vi "Actor Core.vi"(8 "error in":errorcluster, 11 "Nested in":refnum<class "UI Actor.lvclass">) -> (0 "error out":errorcluster, 3 "Actor out":refnum<class "Actor.lvclass">)   [LabVIEW 2020, in "UI Actor.lvlib" / "UI Actor.lvclass"]
doc: "(<B>Filename</B>: Actor Framework.lvlib:Actor.lvclass:Actor Core.vi)\n\nReceives messages to the actor, reacts to them, and initiates any error handling that may shut the actor down.\n\nDescendant classes may override this VI to append parallel tasks for the actor to complete while it handles messages. Overrides use the Call Parent Method node."
uses:
  UI Actor.lvclass
  C:/Program Files (x86)/National Instruments/LabVIEW 2020/vi.lib/ActorFramework/Actor/Actor.lvclass
  <vilib>/ActorFramework/Actor/Actor.lvclass
  <vilib>/ActorFramework/Actor/Actor.lvclass/Actor.ctl
  <vilib>/ActorFramework/Message Enqueuer/Message Enqueuer.lvclass/Message Enqueuer.ctl
  UI Actor.lvclass/UI Actor.ctl
  UI Actor Messages/Set Com Port Msg/Set Com Port Msg.lvclass/Set Com Port Msg.ctl
  UI Actor Messages/Read ADC_UI Actor Msg/Read ADC_UI Actor Msg.lvclass/Read ADC_UI Actor Msg.ctl
  UI Actor Messages/Get Port Status_UI Actor Msg/Get Port Status_UI Actor Msg.lvclass/Get Port Status_UI Actor Msg.ctl
  UI Actor Messages/Set Port Status_UI Actor Msg/Set Port Status_UI Actor Msg.lvclass/Set Port Status_UI Actor Msg.ctl
  UI Actor Messages/Get Pin Status_UI Actor Msg/Get Pin Status_UI Actor Msg.lvclass/Get Pin Status_UI Actor Msg.ctl
  UI Actor Messages/Set Pin Status_UI Actor Msg/Set Pin Status_UI Actor Msg.lvclass/Set Pin Status_UI Actor Msg.ctl
  UI Actor Messages/Set CH Msg/Set CH Msg.lvclass/Set CH Msg.ctl
  UI Actor Messages/Set Pin Msg/Set Pin Msg.lvclass/Set Pin Msg.ctl
  UI Actor Messages/Set valor PIN Msg/Set valor PIN Msg.lvclass/Set valor PIN Msg.ctl
  <vilib>/ActorFramework/Message Enqueuer/Init from Existing Queue.vi
  <vilib>/ActorFramework/Message Enqueuer/Enqueue.vi
  <vilib>/ActorFramework/Stop Msg/Stop Msg.lvclass
  C:/Program Files (x86)/National Instruments/LabVIEW 2020/vi.lib/ActorFramework/Message/Message.lvclass
  UI Actor Messages/Set Com Port Msg/Set Com Port Msg.lvclass
  UI Actor Messages/Read ADC_UI Actor Msg/Read ADC_UI Actor Msg.lvclass
  UI Actor Messages/Get Port Status_UI Actor Msg/Get Port Status_UI Actor Msg.lvclass
  UI Actor Messages/Set Port Status_UI Actor Msg/Set Port Status_UI Actor Msg.lvclass
  UI Actor Messages/Get Pin Status_UI Actor Msg/Get Pin Status_UI Actor Msg.lvclass
  UI Actor Messages/Set Pin Status_UI Actor Msg/Set Pin Status_UI Actor Msg.lvclass
  UI Actor Messages/Set CH Msg/Set CH Msg.lvclass
  UI Actor Messages/Set Pin Msg/Set Pin Msg.lvclass
  UI Actor Messages/Set valor PIN Msg/Set valor PIN Msg.lvclass
  <vilib>/ActorFramework/Message Priority Queue/Priority Enqueue.vi
  <vilib>/Instr/_visa.llb/VISA Configure Serial Port (Instr).vi
  <vilib>/ActorFramework/Message Enqueuer/Message Enqueuer.lvclass
panel:
  in  "Byte 0":string(combo)
  in  "Byte 1":string(combo)
  in  "Valor pin":string(combo)
  in  "PIN":i32
  in  "CH":i32
  out "Display":string
  in  "Set Pin Status":bool
  in  "Get Pin Status":bool
  in  "Set Port Status":bool
  in  "Get Port Status":bool
  in  "Read ADC":bool
  in  "VISA":refnum<visa-resource-name>
  in  "OK Button":bool
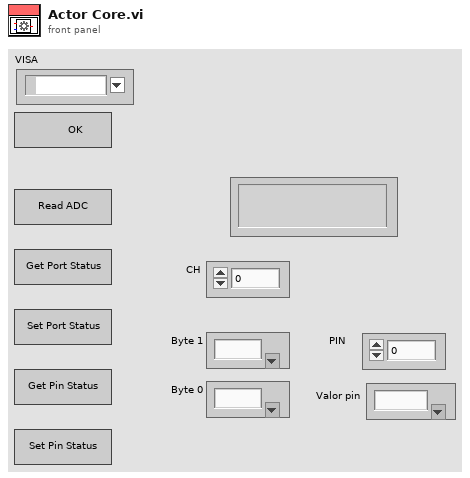
[diagram p1: front panel]
types:
  T1 = cluster{"Stop":refnum<user-event>, "Display":refnum<user-event>}
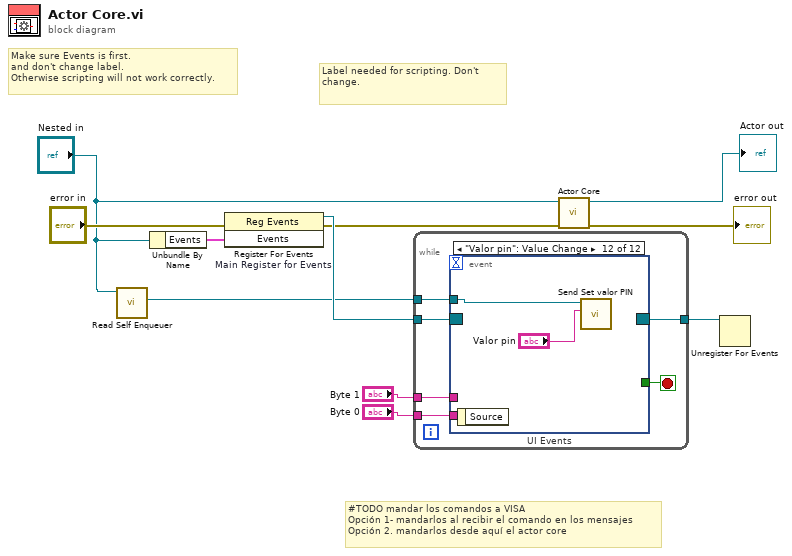
[diagram p0: block diagram]
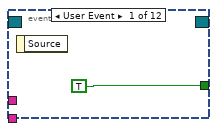
[diagram p2: hidden frame]
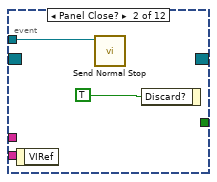
[diagram p3: hidden frame]
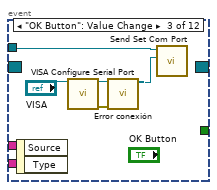
[diagram p4: hidden frame]
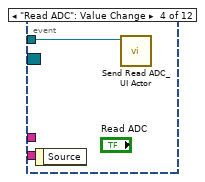
[diagram p5: hidden frame]
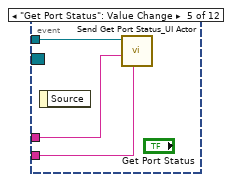
[diagram p6: hidden frame]
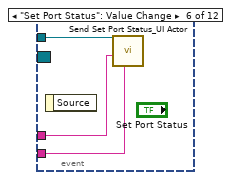
[diagram p7: hidden frame]
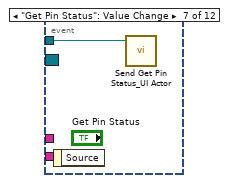
[diagram p8: hidden frame]
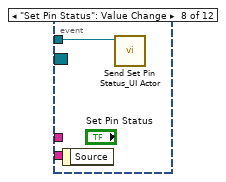
[diagram p9: hidden frame]
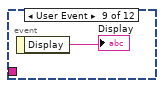
[diagram p10: hidden frame]
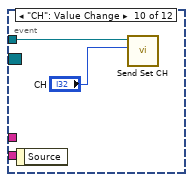
[diagram p11: hidden frame]
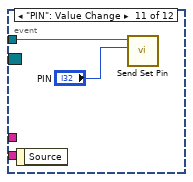
[diagram p12: hidden frame]
diagram:
  # "#TODO mandar los comandos a VISA\nOpción 1- mandarlos al recibir el comando en los mensajes\nOpción 2. mandarlos desde aquí el actor core"
  # "Label needed for scripting. Don't change."
  # "Make sure Events is first.\nand don't change label.\nOtherwise scripting will not work correctly."
  n1 = call <vilib>:"Read Self Enqueuer.vi"("Actor"="Nested in") -> ("Self Enqueuer"=w6:refnum<class "Message Enqueuer.lvclass">)  [unwired: 10 in]
  n2 = Unbundle By Name("Nested in") -> ("Events"=w8:T1)
  n3 = register-events "Main Register for Events"(error in="error in", w8) -> (reference out=w9:refnum<event-registration>, error out=w4:errorcluster)  [unwired: 1 in]
  n4 = while {
    tunnel: w9 -> [w17]
    tunnel: [w15] -> w7
    tunnel: w6 -> [w14]
    tunnel: "Byte 1" -> [w13]
    tunnel: "Byte 0" -> [w12]
    stop <- w16 stop-if-true
    n5 = event "UI Events" shown="[11] \"Valor pin\": Value Change" {
      selector: w17 -> [_ _ _ _ _ _ _ _ _ _ _ _]
      dyn-events: [_ _ _ _ _ _ _ _ _ _ _ _] -> w15
      timeout: _ -> [_ _ _ _ _ _ _ _ _ _ _ _]
      tunnel: [TRUE _ _ _ _ _ _ _ _ _ _ _] -> w16
      tunnel: w14 -> [_ w19 w25 w26 w29 w32 w33 w34 _ w37 w39 w41]
      tunnel: w13 -> [_ _ _ _ w28 w31 _ _ _ _ _ _]
      tunnel: w12 -> [_ _ _ _ w27 w30 _ _ _ _ _ _]
      event User Event {
        n6 = event-data() -> ()  [unwired: 1 in, 1 out]
      }
      event Panel Close? {
        n7 = event-data() -> ()  [unwired: 1 in, 1 out]
        n8 = call <vilib>:"Send Normal Stop.vi"("Message Enqueuer"=w19) -> ()  [unwired: 10 in, 1 out]
        n9 = event-data("Discard?"=TRUE) -> ()  [unwired: 1 in, 1 out]
      }
      event "OK Button": Value Change {
        n10 = event-data() -> ()  [unwired: 1 in, 2 out]
        n11 = call-poly "VISA Configure Serial Port"("VISA resource name"="VISA") -> ("VISA resource name out"=w22:refnum<visa-resource-name>, "error out"=w23:errorcluster)  [unwired: 13 in]
        n12 = call "Error conexión.vi"("error in (no error)"=w23, "VISA Refnum in"=w22) -> ("VISA Refnum out"=w21:refnum<visa-resource-name>)  [unwired: 9 in]
        n13 = call "Send Set Com Port.vi"("VISA resource name"=w21, "Message Enqueuer"=w25) -> ()  [unwired: 8 in, 2 out]
      }
      event "Read ADC": Value Change {
        n14 = event-data() -> ()  [unwired: 1 in, 1 out]
        n15 = call "Send Read ADC_UI Actor.vi"("Message Enqueuer"=w26) -> ()  [unwired: 9 in, 2 out]
      }
      event "Get Port Status": Value Change {
        n16 = event-data() -> ()  [unwired: 1 in, 1 out]
        n17 = call "Send Get Port Status_UI Actor.vi"("Byte 0"=w27, "Byte 1"=w28, "Message Enqueuer"=w29) -> ()  [unwired: 7 in, 2 out]
      }
      event "Set Port Status": Value Change {
        n18 = event-data() -> ()  [unwired: 1 in, 1 out]
        n19 = call "Send Set Port Status_UI Actor.vi"("Byte 0"=w30, "Byte 1"=w31, "Message Enqueuer"=w32) -> ()  [unwired: 7 in, 2 out]
      }
      event "Get Pin Status": Value Change {
        n20 = event-data() -> ()  [unwired: 1 in, 1 out]
        n21 = call "Send Get Pin Status_UI Actor.vi"("Message Enqueuer"=w33) -> ()  [unwired: 9 in, 2 out]
      }
      event "Set Pin Status": Value Change {
        n22 = event-data() -> ()  [unwired: 1 in, 1 out]
        n23 = call "Send Set Pin Status_UI Actor.vi"("Message Enqueuer"=w34) -> ()  [unwired: 9 in, 2 out]
      }
      event User Event {
        n24 = event-data() -> ("Display"=→"Display":string)  [unwired: 1 in]
      }
      event "CH": Value Change {
        n25 = event-data() -> ()  [unwired: 1 in, 1 out]
        n26 = call "Send Set CH.vi"("CH"="CH", "Message Enqueuer"=w37) -> ()  [unwired: 8 in, 2 out]
      }
      event "PIN": Value Change {
        n27 = event-data() -> ()  [unwired: 1 in, 1 out]
        n28 = call "Send Set Pin.vi"("PIN"="PIN", "Message Enqueuer"=w39) -> ()  [unwired: 8 in, 2 out]
      }
      event "Valor pin": Value Change {
        n29 = event-data() -> ()  [unwired: 1 in, 1 out]
        n30 = call "Send Set valor PIN.vi"("Valor pin"="Valor pin", "Message Enqueuer"=w41) -> ()  [unwired: 8 in, 2 out]
      }
    }
  }
  n31 = call-parent "Actor Core.vi"("error in"=w4, "Actor in"="Nested in") -> ("error out"=→"error out":errorcluster, "Actor out"=→"Actor out":refnum<class "Actor.lvclass">)  [unwired: 8 in]
  n32 = Unregister For Events(event registration refnum=w7) -> ()  [unwired: 1 in, 1 out]
